vi "SHCHA Specific Heat Capacity of Humid Air (KJ to Kg K).vi"(1 "Gas Presure":dbl[unit]=80000.0 min=80000.0 max=120000.0, 2 "Tceg":dbl[unit], 3 "RH":dbl) -> (0 "SHCHA":dbl[unit])   [LabVIEW 2018]
panel:
  out "SHCHA\nSpecific Heat Capacity of Humid Air\nSHCHA=SHCDA*(1+(SHCWV-1)*HR)":dbl[unit](knob)
  out "Temprature Of Input Air\nKelvin Degree":dbl[unit](slide) scale=273.0..373.0
  out "Tk":dbl[unit]
  out "Temprature Of Input Air\nCentigrade Degree":dbl[unit](slide) scale=0.0..100.0
  out "Humidity of Input Air":dbl(knob) scale=0.0..100.0
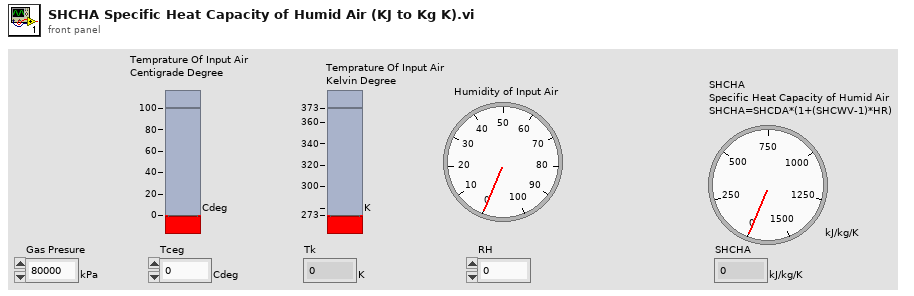
[diagram p1: front panel]
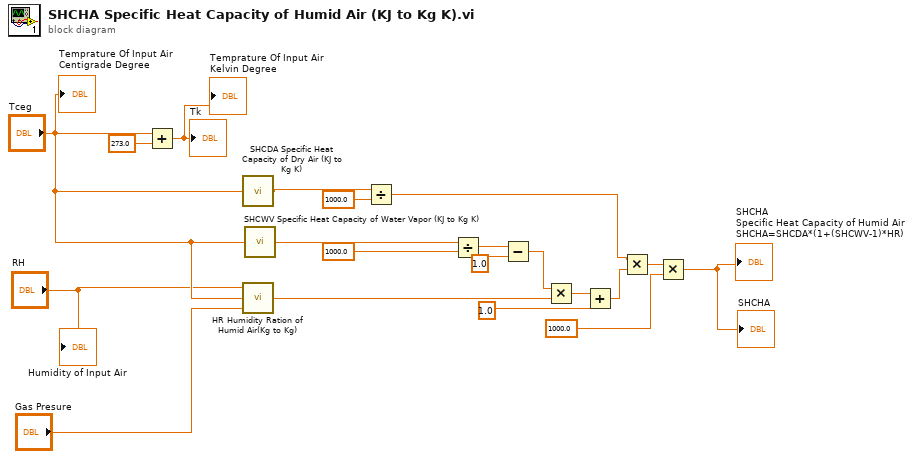
[diagram p0: block diagram]
diagram:
  n1 = Add(x="Tceg", y=dbl[unit] 273.0) -> (x+y=→"Tk" →"Temprature Of Input Air\nKelvin Degree":dbl[unit])
  n2 = call "SHCDA Specific Heat Capacity of Dry Air (KJ to Kg K).vi"("Tceg"="Tceg") -> ("SHCDA"=w9:dbl[unit])
  n3 = call "HR Humidity Ration of Humid Air(Kg to Kg).vi"("Gas Presure"="Gas Presure", "Tceg"="Tceg", "RH"="RH") -> ("HR"=w4:dbl)
  n4 = call "SHCWV Specific Heat Capacity of Water Vapor (KJ to Kg K).vi"("Tceg"="Tceg") -> ("SHCWV"=w11:dbl[unit])
  n5 = Divide(x=w9, y=1000.0) -> (x/y=w8:dbl[unit])
  n6 = Divide(x=w11, y=dbl[unit] 1000.0) -> (x/y=w13:dbl)
  n7 = Subtract(x=w13, y=1.0) -> (x-y=w18:dbl)
  n8 = Multiply(x=w18, y=w4) -> (x*y=w17:dbl)
  n9 = Add(x=w17, y=1.0) -> (x+y=w15:dbl)
  n10 = Multiply(x=w8, y=w15) -> (x*y=w7:dbl[unit])
  n11 = Multiply(x=w7, y=1000.0) -> (x*y=→"SHCHA\nSpecific Heat Capacity of Humid Air\nSHCHA=SHCDA*(1+(SHCWV-1)*HR)" →"SHCHA":dbl[unit])
  "Humidity of Input Air" <- "RH"
  "Temprature Of Input Air\nCentigrade Degree" <- "Tceg"
